vi "Grab images from pco.edge or pco.pixelfly CL with soft ROI.vi"() -> ()   [LabVIEW 2015]
doc: "A short program to demonstrate the fundamentals of control and image acquision with the pco.camera series. The program records a sequence of images, with \"live\" updating, while the \"Record\" button is on. Use ctrl-H for more help on the individual controls and indicators."
panel:
  out "bClose":bool
  in  "Quit":bool
  out "BufNr1":i16
  out "BufNr0":i16
  in  "bUseBuffer1":bool
  in  "bUseBuffer0":bool
  in  "ROIX1":u16=1 min=1
  in  "ROIY1":u16=1 min=1
  in  "ROIY0":u16=1 min=1
  in  "ROIX0":u16=1 min=1
  out "Bits/pixel":u16
  in  "Record":bool
  in  "DelayTimeBase":u16(ring)=2 items=["nanoseconds", "microseconds", "milliseconds"]
  in  "ExposureTimeBase":u16(ring)=2 items=["nanoseconds", "microseconds", "milliseconds"]
  in  "Exposure":u32=10
  in  "Delay":u32
  in  "Rate":i32(ring)
  out "Image":u16[][](graph)
  in  "TriggerMode":u16(ring) items=["Auto", "Software", "External sequence start ", "External exposure control"]
  # "A short program to demonstrate the fundamentals of control and image acquision with the pco.camera series. The program records a sequence of images, with \"live\" updating, while the \"Record\" button is on.  Use ctrl-H for more help on the individual controls and indicators."
  # "pco.labview"
  # "1) Setup camera:"
  # "2) Record  images:"
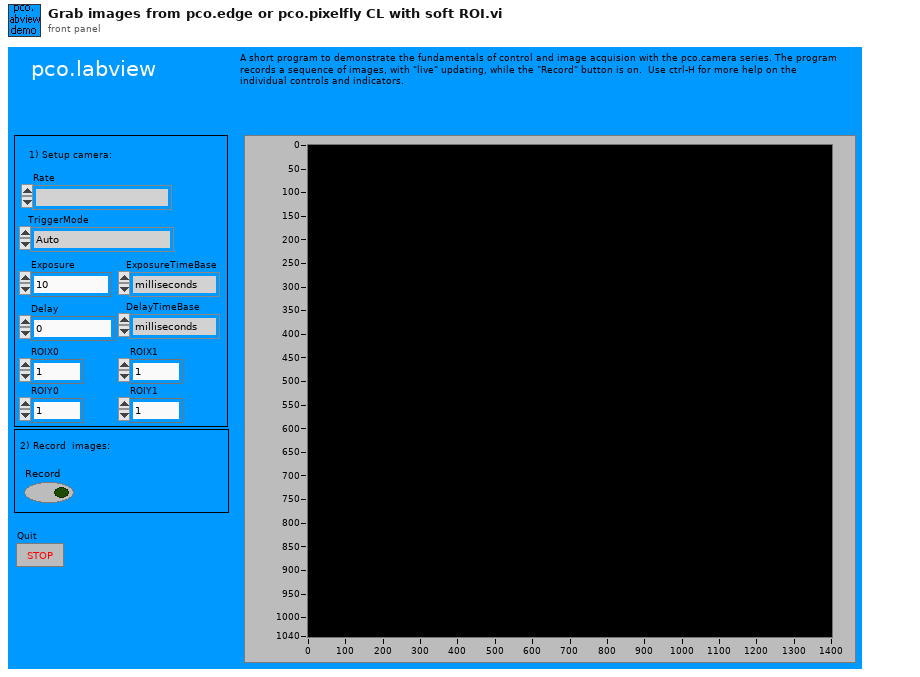
[diagram p1: front panel]
types:
  T1 = cluster{"Size":u16, "InterfaceType":u16, "Camera Number":u16, "CameraNumAtInterface":u16, "OpenFlags":u16[], "OpenDWFlags":u32[], "OpenPtrs":u32[]}
  T2 = cluster{"SSize":u16, "CamType":u16, "CamsSubType":u16, "SerialNumber":u32, "HWVersion":u32, "FWVersion ":u32, "InterfaceType":u16, "HardwareVersions":cluster{"Board":u16, cluster{"string":string, "BatchNumber":u16, "MinorRevision":u8, "MajorRevision":u8, "Variant":u16}[]}, "FirmwareVersions":cluster{"DeviceNum":u16, cluster{"string":string, "MinorRevision":u8, "MajorRevision":u8, "Variant":u16}[]}}
  T3 = cluster{"Size":u16, "SensorTypeDESC":u16, "SensorSubtypeDESC":u16, "MaxHorizontalResStdDESC":u16, "MaxVerticalResStdDESC":u16, "MaxHorizontalResExtDESC":u16, "MaxVerticalResExtDESC":u16, "DynResDESC":u16, "MaxBinHorzDESC":u16, "BinHorzStepDESC":bool, "MaxBinVertDESC":u16, "BinVertStepDESC":bool, "ROIHorzStepDESC":u16, "ROIVertStepDESC":u16, "NumADCDESC":u16, "IRDESC":bool, "MinDelayDESC":u32, "MaxDelayDESC":u32, "MinDelayStepDESC":u32, "MinExpoDESC":u32, "MaxExpoDESC":u32, "MinExpoStepDESC":u32, "MinDelayIRDESC":u32, "MaxDelayIRDESC":u32, "MinExpoIRDESC":u32, "MaxExpoIRDESC":u32, "TimeTableDESC":bool, "DoubleImageDESC":bool, "MinCoolSetDESC":i16, "MaxCoolSetDESC":i16, "MDefaultCoolSetDESC":i16, "PowerDownModeDESC":bool, "OffsetRegDESC":bool, "ColorPattern":cluster{"UpperLeftColor":u8, "UpperRightColor":u8, "LowerLeftColor":u8, "LowerRightColor":u8}, "PatternTypeDESC":bool, "PixelRates":u32[], "CoversionFactors":u16[], "Reserved":u32[], "GeneralCapabilities":u32, "GeneralCapabilities 2":u32, "Min Size Hor":u16, "Min Size Vert":u16, "Ext Synch Freq":u32[], "Cooling Setpoints":i16[], "Soft ROI Hor Step":u16, "Soft ROI Vert Step":u16}
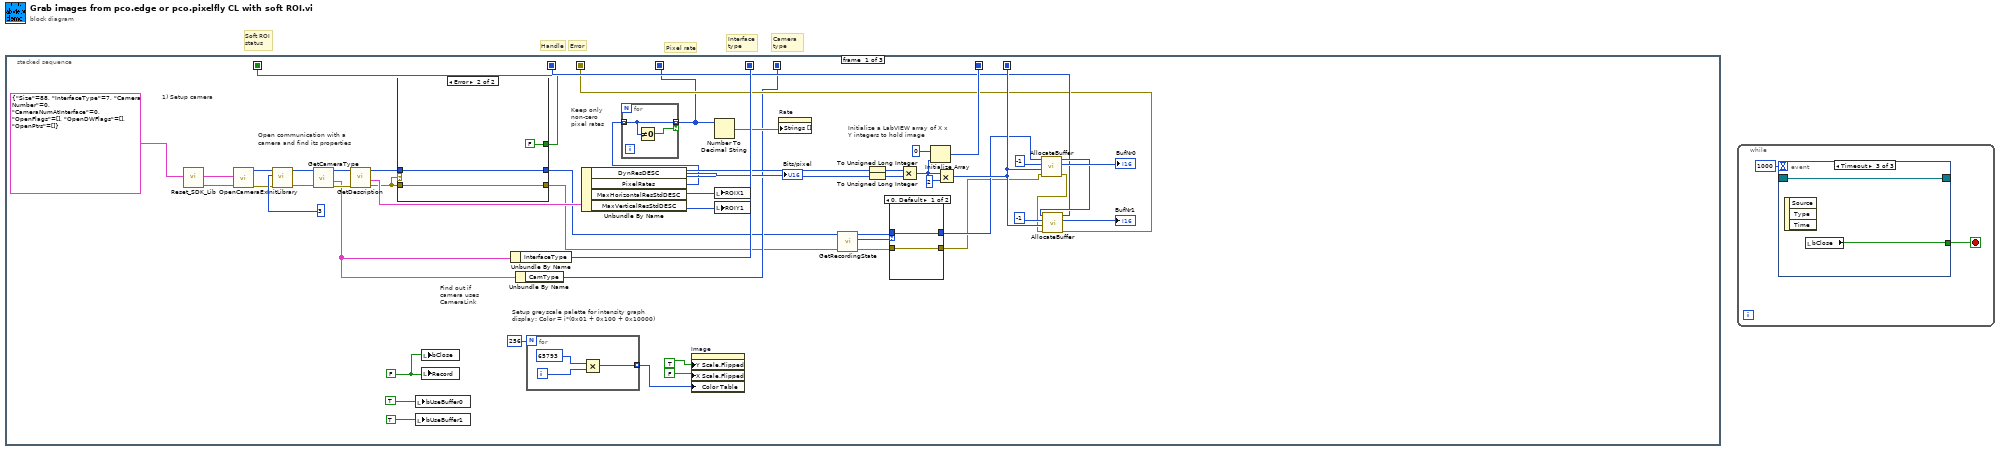
[diagram p0: block diagram]
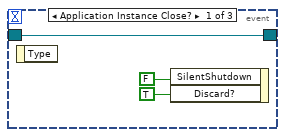
[diagram p2: hidden frame]
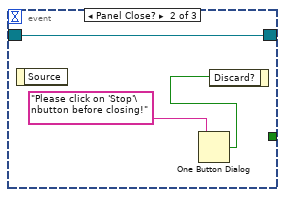
[diagram p3: hidden frame]
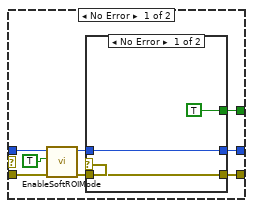
[diagram p4: hidden frame]
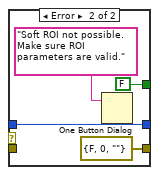
[diagram p5: hidden frame]
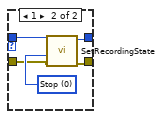
[diagram p6: hidden frame]
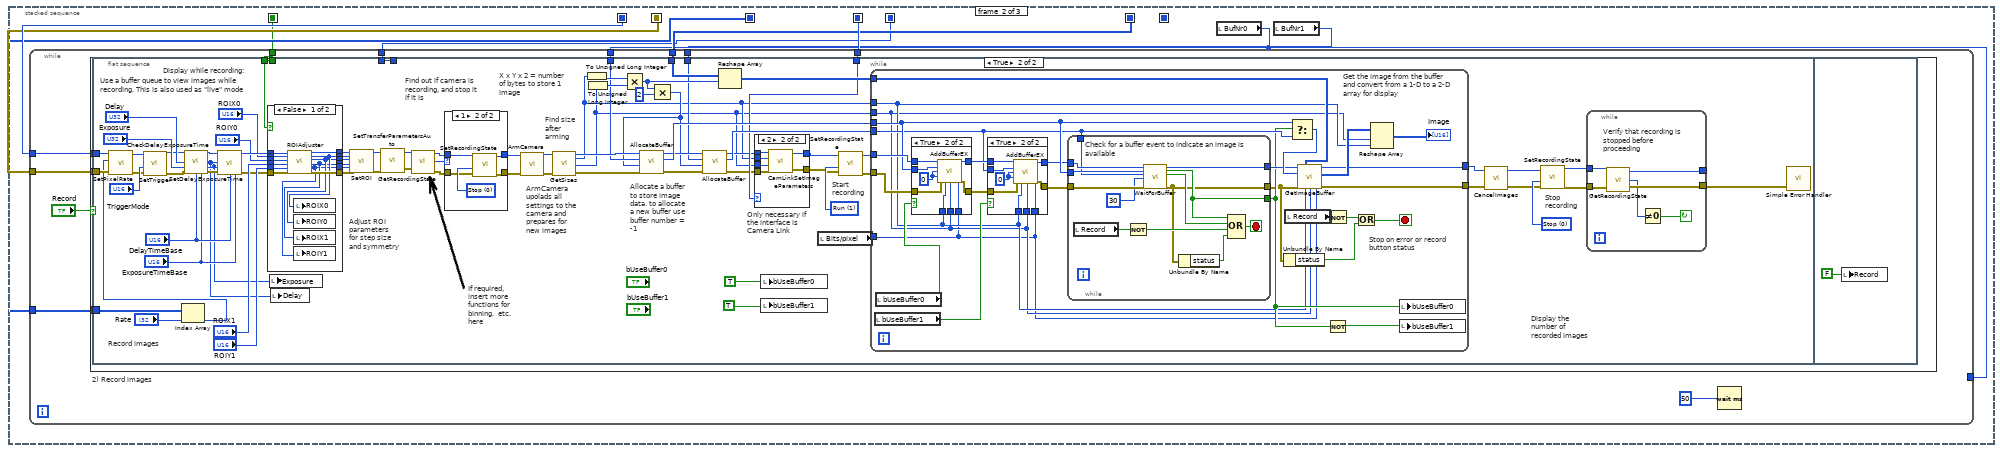
[diagram p7: hidden frame]
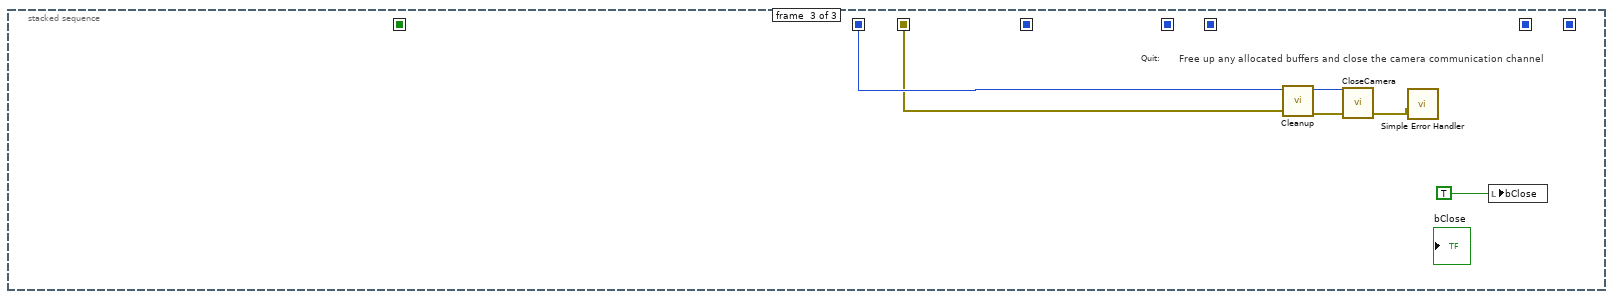
[diagram p14: hidden frame]
diagram:
  # "Soft ROI\nstatus"
  # "Camera type"
  # "Interface type"
  # "Error"
  # "Handle"
  # "Pixel rate"
  n1 = stacked-sequence {
    seq-local: [w45 _ _] -> [_ w87 _]
    seq-local: [w33 _ _] -> [_ _ _]
    seq-local: [w17 _ _] -> [_ w90 w293]
    seq-local: [w16 _ _] -> [_ w89 w292]
    seq-local: [w40 _ _] -> [_ w88 _]
    seq-local: [w5 _ _] -> [_ w84 _]
    seq-local: [w12 _ _] -> [_ w83 _]
    seq-local: [w7 _ _] -> [_ w82 _]
    frame #0 {
      w27 = FALSE ("stop")
      # "Keep only non-zero pixel rates"
      # "1) Setup camera"
      # "Find out if camera uses CameraLink"
      # "Setup greyscale palette for intensity graph display: Color = i*(0x01 + 0x100 + 0x10000)"
      # "Initialize a LabVIEW array of X x Y integers to hold image"
      # "Open communication with a camera and find its properties"
      n2 = call "Reset_SDK_Lib.vi"() -> ("ErrorOut"=w4:errorcluster)  [unwired: 11 in]
      n3 = call "OpenCameraEx.vi"("error in (no error)"=w4, "OpenStructureIn"=T1 {"Size"=88, "InterfaceType"=7, "Camera Number"=0, "CameraNumAtInterface"=0, "OpenFlags"=[], "OpenDWFlags"=[], "OpenPtrs"=[]}) -> ("error out"=w3:errorcluster, "hout"=w1:u64)  [unwired: 2 in, 2 out]
      n4 = call "InitLibrary.vi"("error in (no error)"=w3, "InterfaceType"=u32 3, "ph"=w1) -> ("error out"=w25:errorcluster, "hout"=w24:u64)  [unwired: 7 in]
      n5 = call "GetCameraType.vi"("ph"=w24, "error in (no error)"=w25) -> ("hout"=w42:u64, "CameraType"=w13:T2, "error out"=w41:errorcluster)  [unwired: 1 in, 1 out]
      n6 = call "GetDescription.vi"("ErrorIn"=w41, "ph"=w42) -> ("ErrorOut"=w8:errorcluster, "Description"=w44:T3, "hout"=w11:u64)  [unwired: 2 in, 1 out]
      n7 = case shown="Error" w8 {
        tunnel: w11 -> [w61 w71]
        tunnel: [w57 w71] -> w10
        tunnel: w8 -> [w59 w70]
        tunnel: [w56 w70] -> w9
        tunnel: [w54 FALSE] -> w7
        frame No Error {
          n8 = call "EnableSoftROIMode.vi"("error in (no error)"=w59, "SoftROI"=TRUE, "ph"=w61) -> ("error out"=w55:errorcluster, "hout"=w58:u64)  [unwired: 3 in, 1 out]
          n9 = case shown="No Error" w55 {
            tunnel: w58 -> [w64 w68]
            tunnel: [w64 w68] -> w57
            tunnel: w55 -> [w63 _]
            tunnel: [w63 errorcluster {"status"=FALSE, "code"=0, "source"=""} ("error out")] -> w56
            tunnel: [TRUE FALSE] -> w54
            frame No Error {
            }
            frame Error {
              n10 = One Button Dialog(message="Soft ROI not possible. Make sure ROI parameters are valid.") -> ()  [unwired: 1 in, 1 out]
            }
          }
        }
        frame Error {
        }
      }
      n11 = local write "bUseBuffer0"(TRUE) -> ()
      n12 = local write "bUseBuffer1"(TRUE) -> ()
      n13 = local write "bClose"(w27) -> ()
      n14 = local write "Record"(w27) -> ()
      n15 = Unbundle By Name(w13) -> ("InterfaceType"=w40:u16)
      n16 = Unbundle By Name(w13) -> ("CamType"=w12:u16)
      n17 = for {
        N: 256 -> [_]
        tunnel: [w79] -> w48 mode=indexing
        i -> [w80]
        n18 = Multiply(x=65793, y=w80) -> (x*y=w79:i32)
      }
      n19 = Unbundle By Name(w44) -> ("DynResDESC"=→"Bits/pixel":u16, "PixelRates"=w6:u32[], "MaxHorizontalResStdDESC"=w38:u16, "MaxVerticalResStdDESC"=w37:u16)
      n20 = for {
        tunnel: w6 -> [w53] mode=indexing
        tunnel: [w53] -> w5 mode=indexing if=w52
        n21 = Not Equal To 0?(x=w53) -> (x != 0?=w52:bool)
      }
      n22 = property on="Image" class="IntGraph (strict)"("Y Scale.Flipped"=TRUE, "X Scale.Flipped"=FALSE, "Color Table"=w48) -> ()  [unwired: 2 in, 2 out]
      n23 = Number To Decimal String(number=w5) -> (decimal integer string=w26:string[])  [unwired: 1 in]
      n24 = local write "ROIX1"(w38) -> ()
      n25 = local write "ROIY1"(w37) -> ()
      n26 = property on="Rate" class="Ring (strict)"("Strings []"=w26) -> ()  [unwired: 2 in, 2 out]
      n27 = call "GetRecordingState.vi"("ErrorIn"=w9, "ph"=w10) -> ("ErrorOut"=w20:errorcluster, "Error"=w14:i32, "hout"=w21:u64)  [unwired: 2 in, 1 out]
      n28 = To Unsigned Long Integer(number=w38) -> (unsigned 32bit integer=w35:u32)
      n29 = To Unsigned Long Integer(number=w37) -> (unsigned 32bit integer=w34:u32)
      n30 = case shown="0, Default" w14 {
        tunnel: w21 -> [w73 w77]
        tunnel: w20 -> [w72 w76]
        tunnel: [w73 w75] -> w19
        tunnel: [w72 w74] -> w15
        frame 0, Default {
        }
        frame 1 {
          w78 = u16 0 items=["Stop", "Run"] ("RecordingState")
          n31 = call "SetRecordingState.vi"("ErrorIn"=w76, "RecordingState"=w78, "ph"=w77) -> ("ErrorOut"=w74:errorcluster, "hout"=w75:u64)  [unwired: 2 in, 1 out]
        }
      }
      n32 = Multiply(x=w35, y=w34) -> (x*y=w46:u32)
      n33 = Initialize Array(u16 0 ("Element Data"), w46) -> (w45:u16[])
      n34 = Multiply(x=w46, y=u32 2) -> (x*y=w33:u32)
      n35 = call "AllocateBuffer.vi"("error in (no error)"=w15, "Size"=w33, "BufNr"=i16 -1, "ph"=w19) -> ("error out"=w22:errorcluster, "BufNrOut"=→"BufNr0":i16, "hout"=w18:u64)  [unwired: 2 in, 3 out]
      n36 = call "AllocateBuffer.vi"("error in (no error)"=w22, "Size"=w33, "BufNr"=i16 -1, "ph"=w18) -> ("error out"=w16:errorcluster, "BufNrOut"=→"BufNr1":i16, "hout"=w17:u64)  [unwired: 2 in, 3 out]
    }
    frame #1 {
      n37 = local read "BufNr0"() -> (w86:i16)
      n38 = local read "BufNr1"() -> (w85:i16)
      n39 = while {
        tunnel: w86 -> [_]
        tunnel: w86 -> [w97]
        tunnel: w87 -> [w99]
        tunnel: w88 -> [w100]
        tunnel: w89 -> [w98]
        tunnel: w90 -> [w95]
        tunnel: w85 -> [w96]
        tunnel: w84 -> [w93]
        tunnel: w83 -> [w92]
        tunnel: w82 -> [w91]
        stop <- "Quit" stop-if-true
        n40 = case "2) Record images" shown="True" "Record" {
          tunnel: w95 -> [_ w111]
          tunnel: w98 -> [_ w110]
          tunnel: w100 -> [_ w104]
          tunnel: w99 -> [_ w109]
          tunnel: w97 -> [_ w108]
          tunnel: w96 -> [_ w107]
          tunnel: w93 -> [_ w106]
          tunnel: w92 -> [_ w105]
          tunnel: w91 -> [_ w103]
          frame False {
          }
          frame True {
            n41 = flat-sequence {
              tunnel: w111 -> [w175]
              tunnel: w110 -> [w174]
              tunnel: w109 -> [w171]
              tunnel: w108 -> [w164]
              tunnel: w107 -> [w160]
              tunnel: w106 -> [w147]
              tunnel: w105 -> [_]
              tunnel: w104 -> [w141]
              tunnel: w103 -> [w122]
              frame #0 {
                w186 = u16 1 items=["Stop", "Run"] ("RecordingState")
                w189 = u16 0 items=["Stop", "Run"] ("RecordingState")
                # "Adjust ROI parameters   for step size and symmetry"
                # "Only necessary if the interface is Camera Link"
                # "Display the number of recorded images"
                # "Record images"
                # "Start recording"
                # "Allocate a buffer to store image data. to allocate a new buffer use buffer number = -1"
                # "Find size after arming"
                # "ArmCamera upolads all settings to the camera and prepares for new images"
                # "Find out if camera is recording, and stop it if it is"
                # "If required, insert more functions for binning.  etc. here"
                # "X x Y x 2 = number of bytes to store 1 image"
                # "Stop recording"
                # "Use a buffer queue to view images while recording. This is also used as \"live\" mode"
                # "Display while recording:"
                n42 = Index Array(array=w147, index="Rate") -> (element=w146:u32)
                n43 = call "SetPixelRate.vi"("error in (no error)"=w174, "PixelRate"=w146, "ph"=w175) -> ("error out"=w149:errorcluster, "hout"=w150:u64)  [unwired: 2 in, 1 out]
                n44 = call "SetTrigger.vi"("error in (no error)"=w149, "TriggerMode"="TriggerMode", "ph"=w150) -> ("error out"=w118:errorcluster, "hout"=w119:u64)  [unwired: 2 in, 1 out]
                n45 = call "CheckDelayExposureTime.vi"("ph"=w119, "Delay"="Delay", "Exposure"="Exposure", "error in (no error)"=w118, "DelayTimeBase"="DelayTimeBase", "ExposureTimeBase"="ExposureTimeBase") -> ("hout"=w116:u64, "Delay Out"=w112:u32, "Exposure Out"=w113:u32, "error out"=w117:errorcluster)  [unwired: 4 in, 2 out]
                n46 = call "SetDelayExposureTime.vi"("ph"=w116, "Delay"=w112, "Exposure"=w113, "error in (no error)"=w117, "DelayTimeBase"="DelayTimeBase", "ExposureTimeBase"="ExposureTimeBase") -> ("hout"=w134:u64, "error out"=w124:errorcluster)  [unwired: 7 in, 1 out]
                n47 = case shown="False" w122 {
                  tunnel: w134 -> [w201 w207]
                  tunnel: [w200 w207] -> w133
                  tunnel: "ROIX0" -> [w199 w206]
                  tunnel: "ROIY0" -> [w198 w205]
                  tunnel: "ROIX1" -> [w197 w204]
                  tunnel: "ROIY1" -> [w196 w203]
                  tunnel: [w193 w206] -> w128
                  tunnel: [w192 w205] -> w127
                  tunnel: [w191 w204] -> w126
                  tunnel: [w190 w203] -> w125
                  tunnel: w124 -> [w195 w202]
                  tunnel: [w194 w202] -> w123
                  frame False {
                    n48 = call "ROIAdjuster.vi"("HandleIn"=w201, "ROIXmin"=w199, "ROIYmin"=w198, "ROIXmax"=w197, "ROIYmax"=w196, "ErrorIn"=w195) -> ("hout"=w200:u64, "ROIX0Mod"=w193:u16, "ROIY0Mod"=w192:u16, "ROIX1Mod"=w191:u16, "ROIY1Mod"=w190:u16, "ErrorOut"=w194:errorcluster)  [unwired: 7 in, 1 out]
                    n49 = local write "ROIX0"(w193) -> ()
                    n50 = local write "ROIY0"(w192) -> ()
                    n51 = local write "ROIX1"(w191) -> ()
                    n52 = local write "ROIY1"(w190) -> ()
                  }
                  frame True {
                  }
                }
                n53 = local write "Exposure"(w113) -> ()
                n54 = local write "Delay"(w112) -> ()
                n55 = call "SetROI.vi"("ph"=w133, "ROIX0"=w128, "ROIY0"=w127, "ROIX1"=w126, "ROIY1"=w125, "error in (no error)"=w123) -> ("hout"=w145:u64, "error out"=w144:errorcluster)  [unwired: 12 in]
                n56 = call "SetTransferParametersAuto.vi"("error in (no error)"=w144, "ph"=w145) -> ("error out"=w143:errorcluster, "hout"=w142:u64)  [unwired: 2 in, 1 out]
                n57 = call "GetRecordingState.vi"("ErrorIn"=w143, "ph"=w142) -> ("ErrorOut"=w183:errorcluster, "RecordingState"=w185:u16, "hout"=w184:u64)  [unwired: 2 in, 1 out]
                n58 = case shown="1" w185 {
                  tunnel: w184 -> [w285 w289]
                  tunnel: w183 -> [w284 w288]
                  tunnel: [w285 w287] -> w182
                  tunnel: [w284 w286] -> w181
                  frame 0, Default {
                  }
                  frame 1 {
                    w290 = u16 0 items=["Stop", "Run"] ("RecordingState")
                    n59 = call "SetRecordingState.vi"("ErrorIn"=w288, "RecordingState"=w290, "ph"=w289) -> ("ErrorOut"=w286:errorcluster, "hout"=w287:u64)  [unwired: 2 in, 1 out]
                  }
                }
                n60 = call "ArmCamera.vi"("error in (no error)"=w181, "ph"=w182) -> ("error out"=w179:errorcluster, "hout"=w180:u64)  [unwired: 1 in, 1 out]
                n61 = call "GetSizes.vi"("ph"=w180, "ErrorIn"=w179) -> ("hout"=w176:u64, "XResAct"=w136:u16, "YResAct"=w135:u16, "ErrorOut"=w178:errorcluster)  [unwired: 11 in, 3 out]
                n62 = To Unsigned Long Integer(number=w136) -> (unsigned 32bit integer=w165:u32)
                n63 = To Unsigned Long Integer(number=w135) -> (unsigned 32bit integer=w166:u32)
                n64 = Multiply(x=w165, y=w166) -> (x*y=w167:u32)
                n65 = Multiply(x=w167, y=u32 2) -> (x*y=w161:u32)
                n66 = call "AllocateBuffer.vi"("error in (no error)"=w178, "Size"=w161, "BufNr"=w164, "ph"=w176) -> ("error out"=w163:errorcluster, "BufNrOut"=w168:i16, "hout"=w162:u64)  [unwired: 2 in, 3 out]
                n67 = call "AllocateBuffer.vi"("error in (no error)"=w163, "Size"=w161, "BufNr"=w160, "ph"=w162) -> ("error out"=w138:errorcluster, "BufNrOut"=w159:i16, "hout"=w140:u64)  [unwired: 2 in, 3 out]
                n68 = Reshape Array(w171, w167) -> (w170:u16[])
                n69 = case shown="2" w141 {
                  tunnel: w140 -> [w209 w215]
                  tunnel: [w209 w214] -> w139
                  tunnel: w138 -> [w208 w213]
                  tunnel: [w208 w212] -> w137
                  tunnel: w136 -> [_ w211]
                  tunnel: w135 -> [_ w210]
                  frame 0, Default {
                  }
                  frame 2 {
                    n70 = call "CamLinkSetImageParameters.vi"("error in (no error)"=w213, "YRes"=w210, "XRes"=w211, "ph"=w215) -> ("error out"=w212:errorcluster, "hout"=w214:u64)  [unwired: 1 out]
                  }
                }
                n71 = local write "bUseBuffer0"(TRUE) -> ()
                n72 = local write "bUseBuffer1"(TRUE) -> ()
                n73 = local read "Bits/pixel"() -> (w154:u16)
                n74 = call "SetRecordingState.vi"("ErrorIn"=w137, "RecordingState"=w186, "ph"=w139) -> ("ErrorOut"=w173:errorcluster, "hout"=w172:u64)  [unwired: 2 in, 1 out]
                n75 = while {
                  tunnel: w168 -> [w228]
                  tunnel: w170 -> [w238]
                  tunnel: w172 -> [w237]
                  tunnel: w135 -> [w217]
                  tunnel: w136 -> [w218]
                  tunnel: w173 -> [w235]
                  tunnel: [w240] -> w153
                  tunnel: [w241] -> w152
                  tunnel: w159 -> [w227]
                  tunnel: w154 -> [w216]
                  stop <- w219 stop-if-true
                  # "Stop on error or record button status"
                  # "Get the image from the buffer and convert from a 1-D to a 2-D array for display"
                  n76 = local read "bUseBuffer1"() -> (w232:bool)
                  n77 = local read "bUseBuffer0"() -> (w233:bool)
                  n78 = case shown="True" w233 {
                    tunnel: [w244 w253] -> w234
                    tunnel: [w243 w252] -> w236
                    tunnel: w228 -> [_ w251]
                    tunnel: w237 -> [w243 w250]
                    tunnel: w216 -> [_ w248]
                    tunnel: w218 -> [_ w247]
                    tunnel: w217 -> [_ w246]
                    tunnel: w235 -> [w244 w245]
                    frame False {
                    }
                    frame True {
                      w249 = i16 0
                      n79 = call "AddBufferEX.vi"("ph"=w250, "BuffNr"=w251, "1stImage"=w249, "LastImage"=w249, "error in (no error)"=w245, "XRes"=w247, "YRes"=w246, "BitPerPixel"=w248) -> ("hout"=w252:u64, "error out"=w253:errorcluster)  [unwired: 5 in, 1 out]
                    }
                  }
                  n80 = case shown="True" w232 {
                    tunnel: [w254 w264] -> w225
                    tunnel: [w255 w263] -> w226
                    tunnel: w227 -> [_ w262]
                    tunnel: w236 -> [w255 w261]
                    tunnel: w216 -> [_ w259]
                    tunnel: w218 -> [_ w258]
                    tunnel: w217 -> [_ w257]
                    tunnel: w234 -> [w254 w256]
                    frame False {
                    }
                    frame True {
                      w260 = i16 0
                      n81 = call "AddBufferEX.vi"("ph"=w261, "BuffNr"=w262, "1stImage"=w260, "LastImage"=w260, "error in (no error)"=w256, "XRes"=w258, "YRes"=w257, "BitPerPixel"=w259) -> ("hout"=w263:u64, "error out"=w264:errorcluster)  [unwired: 5 in, 1 out]
                    }
                  }
                  n82 = while {
                    tunnel: w228 -> [w272]
                    tunnel: w227 -> [w271]
                    tunnel: w226 -> [w274]
                    tunnel: w225 -> [w273]
                    tunnel: [w270] -> w224
                    tunnel: [w266] -> w222
                    tunnel: [w269] -> w223
                    stop <- w275 stop-if-true
                    # "Check for a buffer event to indicate an image is available"
                    n83 = local read "Record"() -> (w277:bool)
                    n84 = Not(x=w277) -> (.not. x?=w276:bool)
                    n85 = call "WaitForBuffer.vi"("ph"=w274, "sBufNr"=w272, "sBufNr 2"=w271, "timeout"=30, "error in (no error)"=w273) -> ("hout"=w270:u64, "Buffer_Ready"=w269:bool, "Buffer_Ready 2"=w268:bool, "error out"=w266:errorcluster)  [unwired: 10 in, 1 out]
                    n86 = Unbundle By Name(w266) -> ("status"=w265:bool)
                    n87 = Compound Arithmetic op=OR(w269, w268, w276, w265) -> (w275:bool)
                  }
                  n88 = Unbundle By Name(w222) -> ("status"=w220:bool)
                  n89 = local read "Record"() -> (w239:bool)
                  n90 = Select(t=w228, s=w223, f=w227) -> (s? t:f=w231:i16)
                  n91 = call "GetImageBuffer.vi"("ph"=w224, "BuffIn"=w238, "BuffNr"=w231, "error in (no error)"=w222, "xRes"=w218, "yRes"=w217, "Bitresolution"=w216) -> ("hout"=w240:u64, "BuffOut"=w242:u16[], "error out"=w241:errorcluster)  [unwired: 5 in, 1 out]
                  n92 = Not(x=w223) -> (.not. x?=w230:bool)
                  n93 = Not(x=w239) -> (.not. x?=w221:bool)
                  n94 = Or(x=w221, y=w220) -> (x .or. y?=w219:bool)
                  n95 = Reshape Array(w242, w217, w218) -> (→"Image":u16[][])
                  n96 = local write "bUseBuffer0"(w223) -> ()
                  n97 = local write "bUseBuffer1"(w230) -> ()
                }
                n98 = call "CancelImages.vi"("error in (no error)"=w152, "ph"=w153) -> ("error out"=w156:errorcluster, "hout"=w155:u64)  [unwired: 1 in, 1 out]
                n99 = call "SetRecordingState.vi"("ErrorIn"=w156, "RecordingState"=w189, "ph"=w155) -> ("ErrorOut"=w187:errorcluster, "hout"=w188:u64)  [unwired: 2 in, 1 out]
                n100 = while {
                  tunnel: [w281] -> w151
                  tunnel: w187 -> [w282]
                  tunnel: w188 -> [w283]
                  tunnel: [w278] -> _
                  stop <- w279 continue-if-true
                  # "Verify that recording is stopped before proceeding"
                  n101 = call "GetRecordingState.vi"("ErrorIn"=w282, "ph"=w283) -> ("ErrorOut"=w281:errorcluster, "RecordingState"=w280:u16, "hout"=w278:u64)  [unwired: 2 in, 1 out]
                  n102 = Not Equal To 0?(x=w280) -> (x != 0?=w279:bool)
                }
                n103 = call <vilib>:"Simple Error Handler.vi"("error in (no error)"=w151) -> ()  [unwired: 4 in, 5 out]
              }
              frame #1 {
                n104 = local write "Record"(FALSE ("Record")) -> ()
              }
            }
          }
        }
        n105 = Wait (ms)(milliseconds to wait=u32 50) -> ()  [unwired: 1 out]
      }
    }
    frame #2 {
      # "Free up any allocated buffers and close the camera communication channel"
      # "Quit:"
      n106 = call "Cleanup.vi"("error in (no error)"=w292, "ph"=w293) -> ("error out"=w294:errorcluster, "hout"=w295:u64)  [unwired: 8 in]
      n107 = call "CloseCamera.vi"("ErrorIn"=w294, "Handle in"=w295) -> ("ErrorOut"=w297:errorcluster)  [unwired: 1 in, 2 out]
      n108 = call <vilib>:"Simple Error Handler.vi"("error in (no error)"=w297) -> ()  [unwired: 4 in, 5 out]
      n109 = local write "bClose"(TRUE) -> ()
    }
  }
  n110 = while {
    stop <- w298 stop-if-true
    n111 = event shown="[2] Timeout" {
      selector: _ -> [w300 w305 w307]
      dyn-events: [w300 w305 w307] -> _
      timeout: 1000 -> [_ _ _]
      tunnel: [_ _ w306] -> w298
      event Application Instance Close? {
        n112 = event-data() -> ()  [unwired: 1 in, 1 out]
        n113 = event-data("SilentShutdown"=FALSE, "Discard?"=TRUE) -> ()  [unwired: 1 in, 1 out]
      }
      event Panel Close? {
        n114 = event-data() -> ()  [unwired: 1 in, 1 out]
        n115 = One Button Dialog(message="Please click on 'Stop'\nbutton before closing!") -> (true=w303:bool)  [unwired: 1 in]
        n116 = event-data("Discard?"=w303) -> ()  [unwired: 1 in, 1 out]
      }
      event Timeout {
        n117 = event-data() -> ()  [unwired: 1 in, 3 out]
        n118 = local read "bClose"() -> (w306:bool)
      }
    }
  }
